vi "ModelSS.vi"() -> ()   [LabVIEW 2011]
uses:
  <vilib>/Simulation/Scripting/Companion Diagram/SimConfigNode/SimParams.ctl
  <vilib>/Simulation/Scripting/Companion Diagram/SimConfigNode/_simSolvers.ctl
  <vilib>/Simulation/Implementation/Shared/SIMSCR Execution Mode.ctl
  <vilib>/Simulation/Param Hierarchy/Typedefs/SIMPH Param Control Actions.ctl
  <vilib>/addons/Control Design/_Model Construction/Data Typedefs.llb/CD Time Info.ctl
  <vilib>/Simulation/Implementation/Shared/NILVSim_FinalizeModel.vi
  <vilib>/Simulation/SignalDisplay/Implementation/NILVSim Time Waveform.llb/SIM Time Waveform (scalar).vi
  <vilib>/Simulation/DataSources/Implementation/NILVSim Step.llb/SIM Step (scalar).vi
  <vilib>/Simulation/ContinuousLinear/Implementation/NILVSim State Space.llb/SIM State Space Distributor (SISO CD).vi
  <vilib>/Simulation/ContinuousLinear/Implementation/NILVSim State Space.llb/SIM State Space Collector (SISO CD).vi
  <vilib>/Simulation/ContinuousLinear/Implementation/NILVSim Transfer Function.llb/SIM Transfer Function Collector (SISO).vi
  <vilib>/Simulation/ContinuousLinear/Implementation/NILVSim Transfer Function.llb/SIM Transfer Function Distributor (SISO).vi
  <vilib>/Simulation/ContinuousLinear/Implementation/NILVSim State Space.llb/SIM State Space Distributor (CD).vi
  <vilib>/Simulation/ContinuousLinear/Implementation/NILVSim State Space.llb/SIM State Space Collector (CD).vi
  <vilib>/Simulation/Implementation/Shared/NILVSim_Manager.vi
  <vilib>/Simulation/Implementation/Shared/NILVSim_ParamChanged.vi
  <vilib>/Simulation/Utility/Implementation/NILVSim Get Time and IsAcceptedStep.vi
  <vilib>/addons/Control Design/_Model Construction/Model Creation.llb/Model Creation SubVI/cd_Create State Space Model.vi
  <vilib>/addons/Control Design/_Dynamic Analysis/Dynamic Analysis.llb/Dynamic Analysis subVI/cd_Stability (State-Space).vi
  <vilib>/addons/Control Design/_Model Conversions/Model Type.llb/Model Conversion SubVI/cd_Convert State-Space to Transfer Function Model.vi
  <vilib>/addons/Control Design/_Utility/Model Viewer.llb/Model Viewer SubVI/cd_Draw Transfer Function Equation (TF).vi
  <vilib>/addons/Control Design/_Time Response Analysis/Time Response.llb/Time Response subVI/cd_Parametric Time Response (SS).vi
  <vilib>/addons/Control Design/_Utility/Model Viewer.llb/Model Viewer SubVI/cd_Draw State-Space Equation (SS).vi
  <vilib>/Simulation/Implementation/Shared/SIM Unbundle Sim Info.vi
  <vilib>/Simulation/Implementation/Shared/NILVSim_GetModelError.vi
  <vilib>/Simulation/Implementation/Shared/SIM Bundle Sim Info.vi
  <vilib>/Simulation/Implementation/Shared/NILVSim_Initialize.vi
  <vilib>/addons/control/pid/pid.llb/PID.vi
  <vilib>/addons/control/pid/pid.llb/PID (DBL).vi
  <vilib>/addons/Control Design/_State Feedback Control/State Feedback Control.llb/CD Pole Placement.vi
  <vilib>/addons/Control Design/_State Feedback Control/State Feedback Control.llb/CD State-Space Controller.vi
  <vilib>/addons/Control Design/_State Feedback Control/State Feedback Control.llb/CD State Regulator.vi
  <vilib>/addons/Control Design/_Time Response Analysis/Time Response.llb/CD Step Response.vi
  <vilib>/addons/Control Design/_Time Response Analysis/Time Response.llb/Time Response subVI/cd_Step Response (State-Space).vi
  <vilib>/Analysis/polynomials.llb/Sort Complex Numbers (obs).vi
  <vilib>/addons/Control Design/_State Feedback Control/State Feedback Control.llb/CD Ackermann.vi
  <vilib>/addons/Control Design/_State Feedback Control/State Feedback Control.llb/CD Linear Quadratic Regulator.vi
  <vilib>/addons/Control Design/_State Feedback Control/State Feedback Control.llb/State Feedback Control SubVis/cd_Linear Quadratic Regulator.vi
  <vilib>/Analysis/baseanly.llb/Dot Product.vi
  <vilib>/Analysis/baseanly.llb/Real Dot Product.vi
  <vilib>/Simulation/Scripting/Companion Diagram/SimConfigNode/SimDog.xnode
  <vilib>/Simulation/Implementation/XNodeFramework/SimXNode/SimX.xnode
  <vilib>/addons/Control Design/_Model Construction/NI_LinSys_Model Creation.lvlib
  <vilib>/addons/Control Design/_Time Response Analysis/NI_CD_Time Response.lvlib
  <vilib>/addons/Control Design/_Utility/NI_CD_Model Viewer.lvlib
  <vilib>/addons/Control Design/_Model Conversions/NI_CD_Model Type.lvlib
  <vilib>/addons/Control Design/_Dynamic Analysis/NI_CD_Dynamic Analysis.lvlib
  <vilib>/addons/Control Design/_Model Construction/Model Typedefs.llb/CD General Elements.ctl
  <vilib>/addons/Control Design/_Model Construction/NI_LinSys_Model Typedefs.lvlib
  <vilib>/addons/Control Design/_Model Construction/Model Typedefs.llb/CD State Space Model (MIMO).ctl
  <vilib>/addons/control/pid/NI_PID_pid.lvlib
  <vilib>/Simulation/ContinuousLinear/Implementation/NILVSim State Space.llb/SIM State Space (CD).vi
  <vilib>/Simulation/ContinuousLinear/Implementation/NILVSim Transfer Function.llb/SIM Transfer Function (SISO).vi
  <vilib>/addons/Control Design/_State Feedback Control/NI_CD_State Feedback Control.lvlib
  <vilib>/Analysis/NI_AALPro.lvlib
  <vilib>/addons/Control Design/_Model Construction/NI_LinSys_Data Typedefs.lvlib
  <vilib>/Analysis/NI_AALBase.lvlib
  <vilib>/Simulation/ContinuousLinear/Implementation/NILVSim State Space.llb/SIM State Space (SISO CD).vi
  <vilib>/Simulation/Implementation/Shared/NI_SIM_Implementation.lvlib
panel:
  out "subarray 2":dbl[](array[numeric])
  in  "Q":dbl[][](array[numeric])=[[1500.0, 0.0], [0.0, 10.0]]
  in  "R":dbl[][](array[numeric])=[[0.0001]]
  out "State Trajectory Graph LQR":cluster{"time":dbl[], dbl[]}[](graph)
  out "Closed-Loop Step Response LQR":cluster{"time":dbl[], dbl[]}[](graph)
  out "Eigenvalues":cdb[](array[numeric]) format="%.2f"
  out "Optimal Gain (K)":dbl[][](array[numeric]) format="%.2f"
  in  "Zdot":dbl=1.0
  in  "Z":dbl=1.0
  out "u":dbl format="%.2f"
  out "State Trajectory Graph":cluster{"time":dbl[], dbl[]}[](graph)
  out "Closed-Loop Step Response":cluster{"time":dbl[], dbl[]}[](graph)
  out "Gain 2":dbl[][](array[numeric]) format="%.2f"
  out "Actual Poles 2":cdb[](array[numeric])=[-4.9512521676495505+0.0i, -3.4076115316471447-10.013861291935113i, -3.4076115316471447+10.013861291935113i] format="%.2f"
  out "Desired Poles":cdb[](array[numeric])=[-4.951252167649562+0.0i, -3.4076115316471642-10.013861291935129i, -3.4076115316471642+10.013861291935129i] format="%.2f"
  out "Actual Poles":cdb[](array[numeric])=[-4.9512521676495505+0.0i, -3.4076115316471447-10.013861291935113i, -3.4076115316471447+10.013861291935113i] format="%.2f"
  out "Gain":dbl[](array[numeric]) format="%.3f"
  in  "Imaginary":dbl(knob)=-10.013861291935129 scale=0.0..-20.0 scale format="%#_4g"
  in  "Real":dbl(knob)=-3.4076115316471642 scale=0.0..-22.0 scale format="%#_4g"
  out "state x(k) 2":dbl[](array[numeric])
  out "output y(k) 3":dbl
  out "Waveform Chart":waveform(dbl)(graph)={"t0"=timestamp(9343.2 s since 1904-01-01), "dt"=1.0, "Y"=[0.2633720690985406]}
  out "state x(k)":dbl[](array[numeric])
  out "output y(k) 2":dbl
  out "Z Process":dbl
  in  "Z":dbl format="%.2f"
  out "Altitude Waveform":waveform(dbl)(graph)={"t0"=timestamp(9343.2 s since 1904-01-01), "dt"=1.0, "Y"=[0.2633720690985406]}
  out "output y(k)":dbl[](array[numeric])
  out "input u(k)":dbl[](array[slide]) scale=0.0..10.0
  out "Stability":T1(ring)=enum."undetermined"
  out "Poles":cdb[](array[numeric]) format="%.2e"
  out "Equation":picture
  out "Quadcopter":picture
  out "Time Response":cluster{"time":dbl[], dbl[]}[](graph) caption="Time Response Graph"
  # "Close-Loop System using Pole-Placement & Ackerman"
  # "State Space"
  # "0.25/S^2"
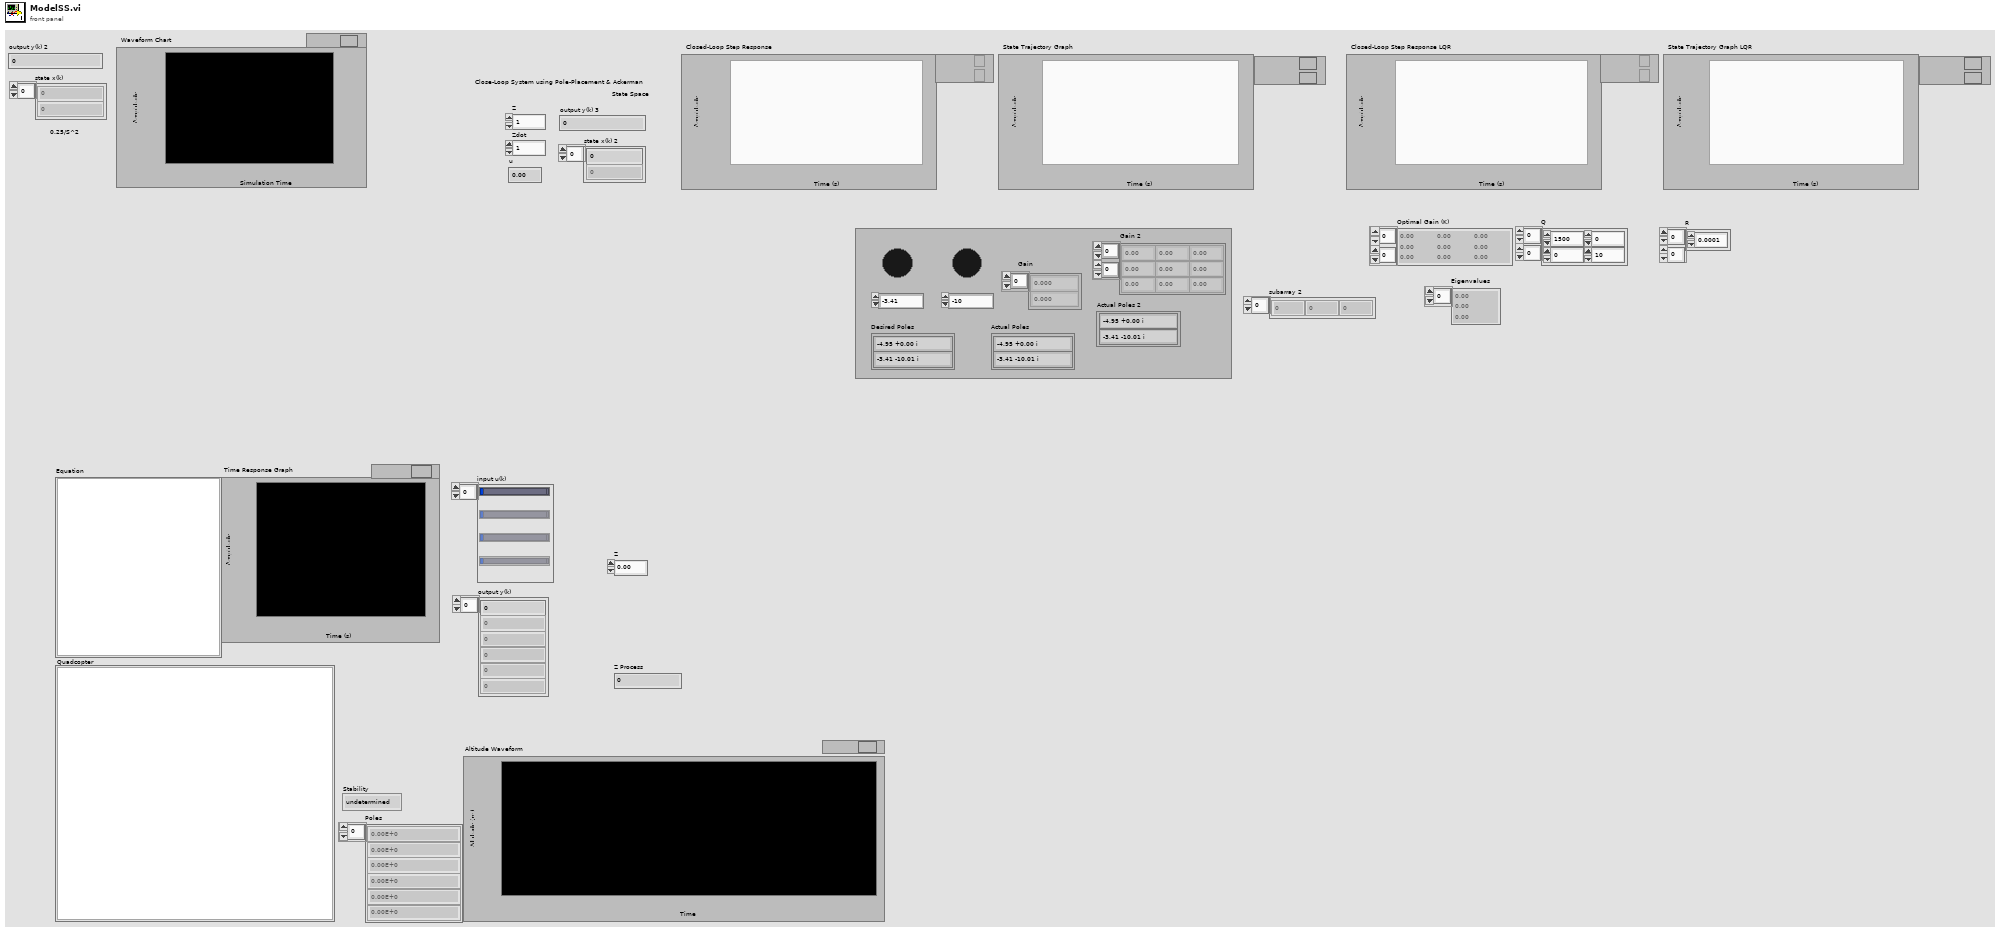
[diagram p1: front panel]
types:
  T1 = enum16{"stable", "marginally stable", "unstable", "undetermined"}
  T2 = typedef "NI_LinSys_Model Typedefs.lvlib/CD State Space Model (MIMO).ctl" = cluster{"properties":T3, "A":dbl[][], "B":dbl[][], "C":dbl[][], "D":dbl[][], "StateNames":string[], "Transport Delay":dbl[][]}
  T3 = typedef "NI_LinSys_Model Typedefs.lvlib/CD General Elements.ctl" = cluster{"Model name":string, "Input names":string[], "Output names":string[], "Input Delays":dbl[], "Output Delays":dbl[], "Sampling Time":dbl, "Notes":string}
  T4 = typedef "NI_LinSys_Model Typedefs.lvlib/CD Transfer Function Model (MIMO).ctl" = cluster{"properties":T3, "transfer function(s)":T5[][]}
  T5 = typedef "NI_LinSys_Model Typedefs.lvlib/CD Transfer Function Model (SISO).ctl" = cluster{"Numerator":dbl[], "Denominator":dbl[], "delay":dbl}
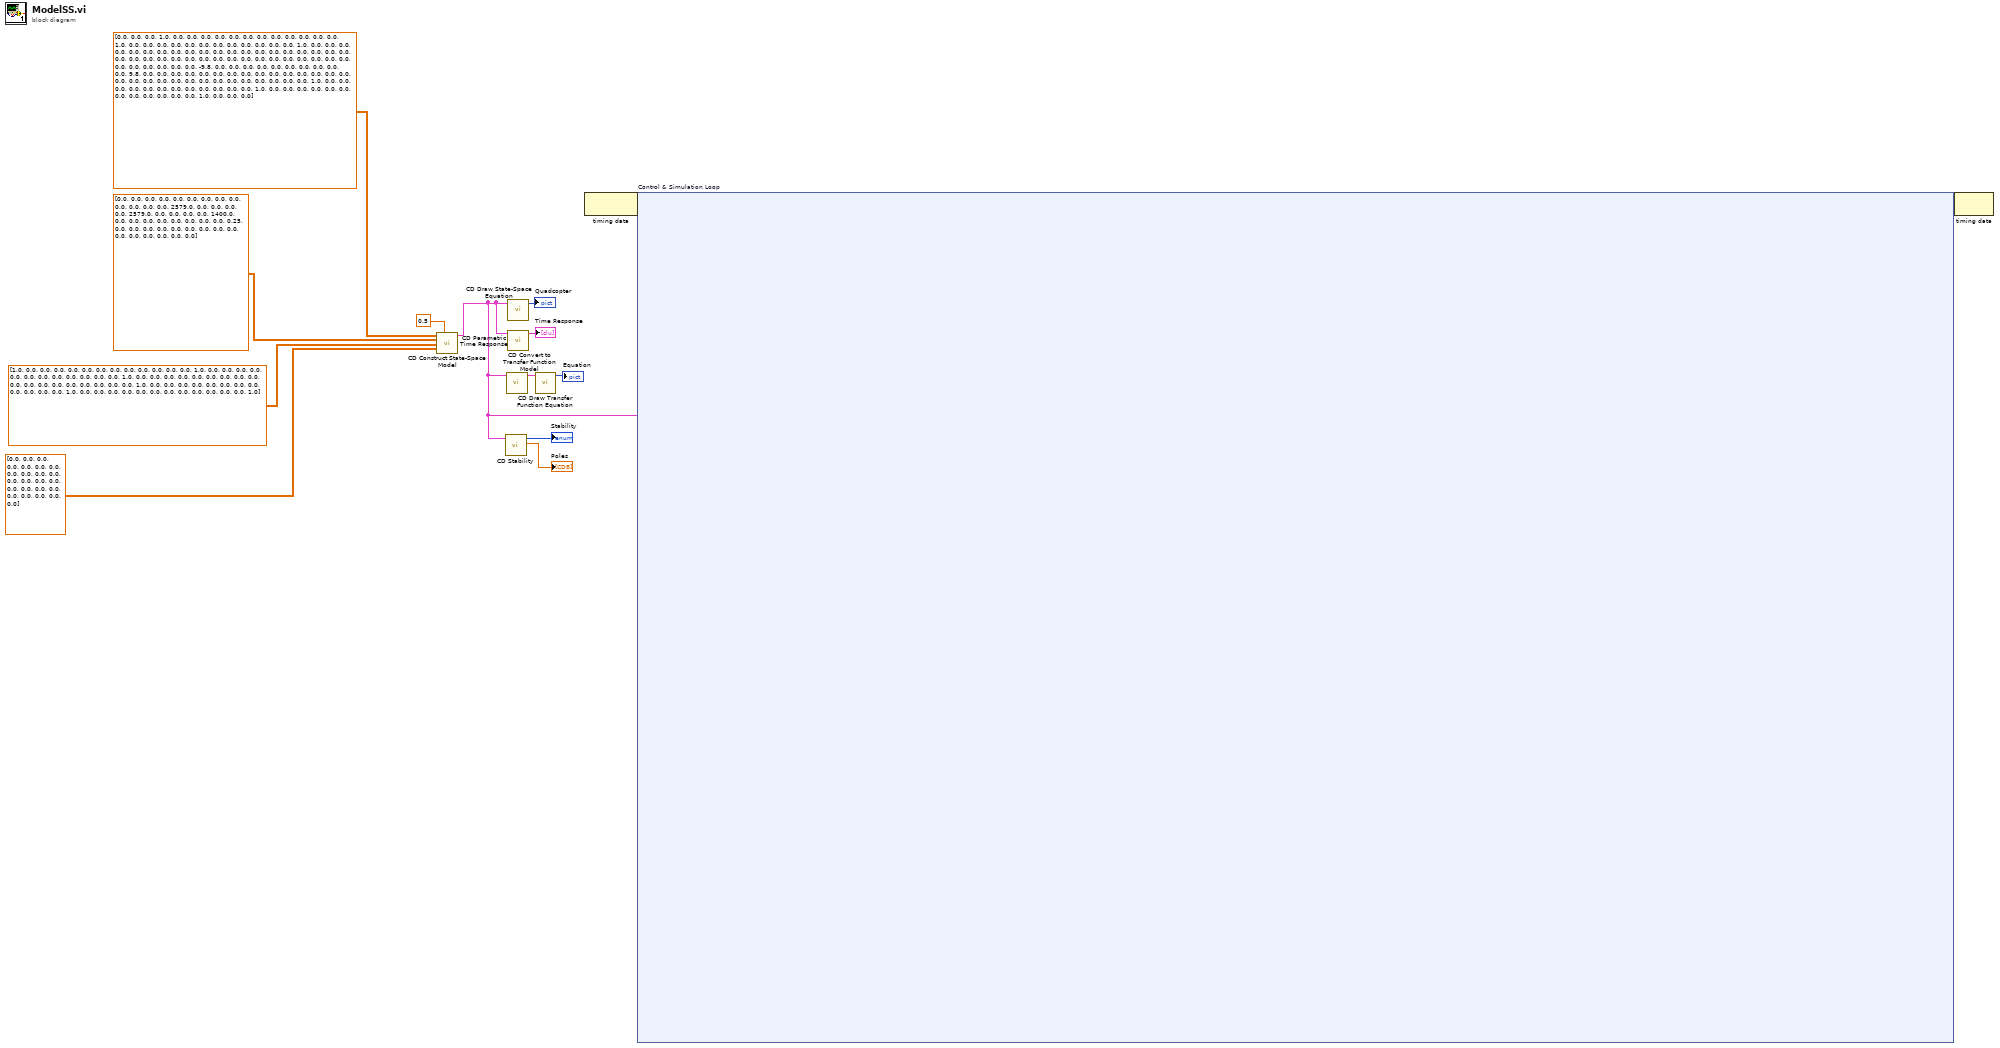
[diagram p0: block diagram]
diagram:
  n1 = call-poly <vilib>:"CD Construct State-Space Model.vi"("A"=dbl[][] [[0.0, 0.0, 0.0, 1.0, 0.0, 0.0, 0.0, 0.0, 0.0, 0.0, 0.0, 0.0], [0.0, 0.0, 0.0, 0.0, 1.0, 0.0, 0.0, 0.0, 0.0, 0.0, 0.0, 0.0], [0.0, 0.0, 0.0, 0.0, 0.0, 1.0, 0.0, 0.0, 0.0, 0.0, 0.0, 0.0], [0.0, 0.0, 0.0, 0.0, 0.0, 0.0, 0.0, 0.0, 0.0, 0.0, 0.0, 0.0], [0.0, 0.0, 0.0, 0.0, 0.0, 0.0, 0.0, 0.0, 0.0, 0.0, 0.0, 0.0], [0.0, 0.0, 0.0, 0.0, 0.0, 0.0, 0.0, 0.0, 0.0, 0.0, 0.0, 0.0], [0.0, -9.8, 0.0, 0.0, 0.0, 0.0, 0.0, 0.0, 0.0, 0.0, 0.0, 0.0], [9.8, 0.0, 0.0, 0.0, 0.0, 0.0, 0.0, 0.0, 0.0, 0.0, 0.0, 0.0], [0.0, 0.0, 0.0, 0.0, 0.0, 0.0, 0.0, 0.0, 0.0, 0.0, 0.0, 0.0], [0.0, 0.0, 0.0, 0.0, 0.0, 0.0, 1.0, 0.0, 0.0, 0.0, 0.0, 0.0], [0.0, 0.0, 0.0, 0.0, 0.0, 0.0, 0.0, 1.0, 0.0, 0.0, 0.0, 0.0], [0.0, 0.0, 0.0, 0.0, 0.0, 0.0, 0.0, 0.0, 1.0, 0.0, 0.0, 0.0]], "Sampling Time (s)"=0.5, "B"=dbl[][] [[0.0, 0.0, 0.0, 0.0], [0.0, 0.0, 0.0, 0.0], [0.0, 0.0, 0.0, 0.0], [0.0, 2579.0, 0.0, 0.0], [0.0, 0.0, 2579.0, 0.0], [0.0, 0.0, 0.0, 1400.0], [0.0, 0.0, 0.0, 0.0], [0.0, 0.0, 0.0, 0.0], [0.25, 0.0, 0.0, 0.0], [0.0, 0.0, 0.0, 0.0], [0.0, 0.0, 0.0, 0.0], [0.0, 0.0, 0.0, 0.0]], "C"=dbl[][] [[1.0, 0.0, 0.0, 0.0, 0.0, 0.0, 0.0, 0.0, 0.0, 0.0, 0.0, 0.0], [0.0, 1.0, 0.0, 0.0, 0.0, 0.0, 0.0, 0.0, 0.0, 0.0, 0.0, 0.0], [0.0, 0.0, 1.0, 0.0, 0.0, 0.0, 0.0, 0.0, 0.0, 0.0, 0.0, 0.0], [0.0, 0.0, 0.0, 0.0, 0.0, 0.0, 0.0, 0.0, 0.0, 1.0, 0.0, 0.0], [0.0, 0.0, 0.0, 0.0, 0.0, 0.0, 0.0, 0.0, 0.0, 0.0, 1.0, 0.0], [0.0, 0.0, 0.0, 0.0, 0.0, 0.0, 0.0, 0.0, 0.0, 0.0, 0.0, 1.0]], "D"=dbl[][] [[0.0, 0.0, 0.0, 0.0], [0.0, 0.0, 0.0, 0.0], [0.0, 0.0, 0.0, 0.0], [0.0, 0.0, 0.0, 0.0], [0.0, 0.0, 0.0, 0.0], [0.0, 0.0, 0.0, 0.0]]) -> ("State-Space Model"=w1:T2)  [unwired: 9 in, 1 out]
  n2 = call-poly <vilib>:"CD Stability.vi"("State-Space Model"=w1) -> ("Poles"=→"Poles":cdb[], "Stability"=→"Stability":T1)  [unwired: 8 in, 1 out]
  n3 = call-poly <vilib>:"CD Convert to Transfer Function Model.vi"("State-Space Model"=w1) -> ("Transfer Function Model"=w7:T4)  [unwired: 9 in, 1 out]
  n4 = call-poly <vilib>:"CD Draw State-Space Equation.vi"("State-Space Model"=w1) -> ("Equation"=→"Quadcopter":picture)  [unwired: 8 in, 2 out]
  n5 = call-poly <vilib>:"CD Parametric Time Response.vi"("State-Space Model"=w1) -> ("Time Response"=→"Time Response":cluster{"time":dbl[], dbl[]}[])  [unwired: 7 in, 3 out]
  n6 = call-poly <vilib>:"CD Draw Transfer Function Equation.vi"("Transfer Function Model"=w7) -> ("Equation"=→"Equation":picture)  [unwired: 8 in, 2 out]
  n7 = node-c288() -> (w3:variant)  [unwired: 1 in]
  n8 = node-c254 "Control & Simulation Loop"(w3, w1) -> (w2:variant)
  n9 = node-c288(w2) -> ()  [unwired: 1 out]
